vi "Query Output State Core.vi"(8 "error in (no error)":errorcluster, 9 "output state (Constant Voltage)":i32(ring) items=["Constant Voltage"=0, "Constant Current"=1, "Unregulated"=4, "Over Voltage"=2, "Over Current"=3], 10 "channel name (\"CHANNEL1\")":string="CHANNEL1", 11 "IVI_DCPwr in":refnum<class "IVI_DCPwr.lvclass">) -> (0 "error out":errorcluster, 2 "in state":bool, 3 "IVI_DCPwr out":refnum<class "IVI_DCPwr.lvclass">)   [LabVIEW 2015, in "IVI_DCPwr.lvlib" / "IVI_DCPwr.lvclass"]
doc: "This VI returns whether the power supply is in a particular output state.\n\nA constant voltage condition occurs when the output voltage is equal to the value of the IviDCPwr>>Basic Operation>>Voltage Level property and the current is less than or equal to the value of the IviDCPwr>>Basic Operation>>Current Limit property.\n\nA constant current condition occurs when the output current is equal to the value of the IviDCPwr>>Basic Operation>>Current Limit property and the IviDCPwr>>Basic Operation>>Current Limit Behavior property is set to IVIDCPWR_VAL_CURRENT_REGULATE.\n\nAn unregulated condition occurs when the output voltage is less than the value of the IviDCPwr>>Basic Operation>>Voltage Level property and the current is less than the value of the IviDCPwr>>Basic Operation>>Current Limit property.\n\nAn over-voltage condition occurs when the output voltage is equal to or greater than the value of the IviDCPwr>>Basic Operation>>OVP Limit property and the IviDCPwr>>Basic Operation>>OVP Enabled property is set to TRUE.\n\nAn over-current condition occurs when the output current is equal to or greater than the value of the IviDCPwr>>Basic Operation>>Current Limit property and the IviDCPwr>>Basic Operation>>Current Limit Behavior property is set to IVIDCPWR_VAL_CURRENT_TRIP. \n\nWhen either an over-voltage condition or an over-current condition occurs, the power supply's output protection disables the output. If the power supply is in an over-voltage or over-current state, it does not produce power until the output protection is reset. The IviDCPwr Reset Output Protection VI resets the output protection. Once the output protection is reset, the power supply resumes generating a power signal."
uses:
  IVI_DCPwr.lvclass
  IVI_DCPwr.lvclass/IVI_DCPwr.ctl
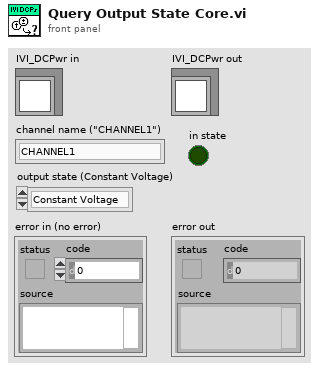
[diagram p1: front panel]
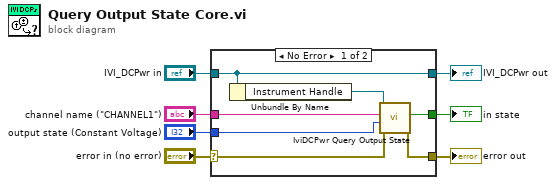
[diagram p0: block diagram]
diagram:
  n1 = case shown="No Error" "error in (no error)" {
    selector: "error in (no error)" -> [w13 w16]
    tunnel: [w12 w16] -> w6
    tunnel: [w8 w15] -> w4
    tunnel: "IVI_DCPwr in" -> [w8 w15]
    tunnel: "channel name (\"CHANNEL1\")" -> [w11 _]
    tunnel: "output state (Constant Voltage)" -> [w10 _]
    tunnel: [w9 _] -> w1
    frame No Error {
      n2 = Unbundle By Name(w8) -> ("Instrument Handle"=w14:refnum<k15>)
      n3 = call <vilib>:"IviDCPwr Query Output State.vi"("error in (no error)"=w13, "output state (Constant Voltage)"=w10, "channel name (\"CHANNEL1\")"=w11, "instrument handle"=w14) -> ("error out"=w12:errorcluster, "in state"=w9:bool)  [unwired: 5 in, 1 out]
    }
    frame Error {
    }
  }
  "error out" <- w6
  "IVI_DCPwr out" <- w4
  "in state" <- w1
